vi "CAPTH-Config.vi"(0 "Datafile":path, 5 "Params":T1={"Stimulus"={"EAR"=enum."RIGHT", "HI FREQ"=18.0, "LO FREQ"=5.0, "FREQ STEP"=8, "Rep Rate (/s)"=20.0, "Alternate Polarity"=TRUE, "# CYCLES"=1, "Duration (ms)"=0.0, "Ramp (ms)"=0.0}, "Response"={"Averages (3dB steps)"=12, "Time Window (ms)"=8.5, "dt (us)"=10.0, "Grass gain"=1000.0, "CRITERION (mV)"=60.0, "CEILING (dB atten)"=6.0, "Use previous"=FALSE, "Save avgs"=FALSE, "Save raw"=FALSE, "Save history"=FALSE, "CEILING (dB SPL)"=6.0}} {"Response"."CRITERION (mV)" format="%.2f"; "Response"."Time Window (ms)" format="%.2f"}, 11 "error in (no error)":errorcluster) -> (3 "IO channels":cluster{"Output":u16, "Input":u16}[](array[cluster]), 4 "Freqs":dbl[](array[numeric]), 6 "runtime":T5, 12 "data":T4(array[cluster]), 13 "active ears":i32[](array[numeric]), 14 "start atten":dbl[](array[numeric]), 15 "error out":errorcluster)   [LabVIEW 2020]
uses:
  Typedefs/CAPTH-Runtime.ctl
  Typedefs/CAPTH-Parameters.ctl
  Typedefs/CAPTH-Stimulus.ctl
  Typedefs/CAPTH-Response.ctl
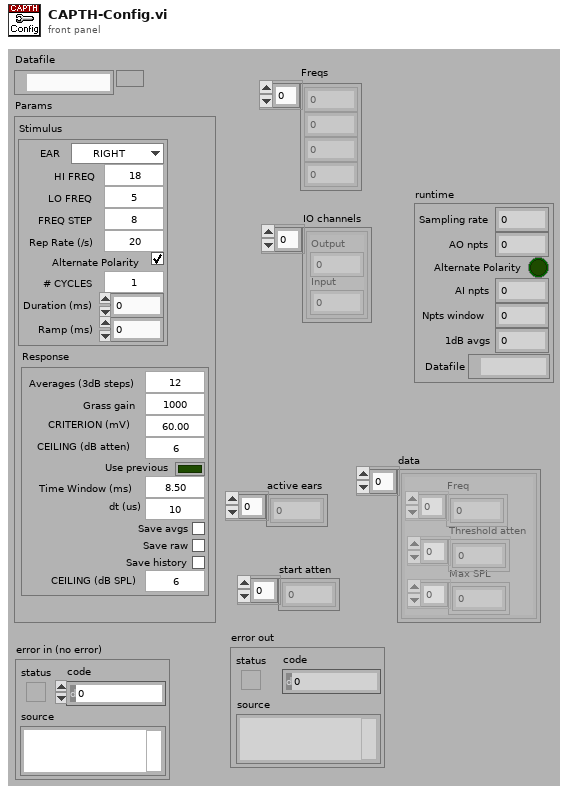
[diagram p1: front panel]
types:
  T1 = typedef "CAPTH-Parameters.ctl" = cluster{"Stimulus":T2, "Response":T3}
  T2 = typedef "CAPTH-Stimulus.ctl" = cluster{"EAR":enum16{"RIGHT", "LEFT\n", "ALTERNATE"}, "HI FREQ":dbl, "LO FREQ":dbl, "FREQ STEP":u8, "Rep Rate (/s)":dbl, "Alternate Polarity":bool, "# CYCLES":u8, "Duration (ms)":dbl, "Ramp (ms)":dbl}
  T3 = typedef "CAPTH-Response.ctl" = cluster{"Averages (3dB steps)":i32, "Time Window (ms)":dbl, "dt (us)":dbl, "Grass gain":dbl, "CRITERION (mV)":dbl, "CEILING (dB atten)":dbl, "Use previous":bool, "Save avgs":bool, "Save raw":bool, "Save history":bool, "CEILING (dB SPL)":dbl}
  T4 = cluster{"Freq":dbl[], "Threshold atten":dbl[], "Max SPL":dbl[]}[]
  T5 = typedef "CAPTH-Runtime.ctl" = cluster{"Sampling rate":dbl, "AO npts":i32, "Alternate Polarity":bool, "AI npts":i32, "Npts window":i32, "1dB avgs":i32, "Datafile":path}
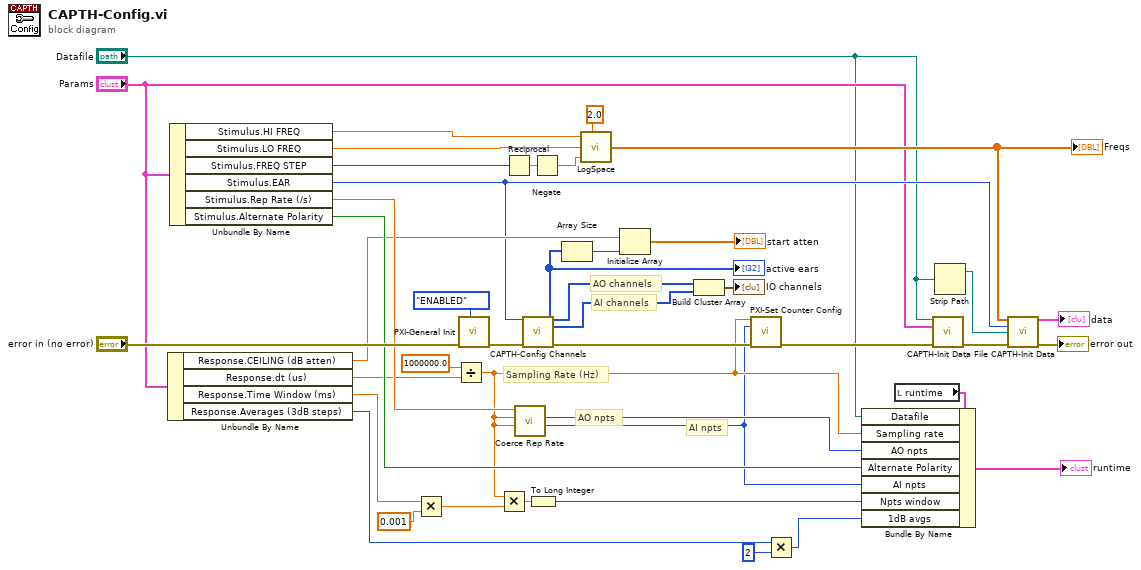
[diagram p0: block diagram]
diagram:
  # "AO channels"
  # "AI channels"
  # "Sampling Rate (Hz)"
  # "AO npts"
  # "AI npts"
  n1 = Unbundle By Name("Params") -> ("Response.CEILING (dB atten)"=w19:dbl, "Response.dt (us)"=w22:dbl, "Response.Time Window (ms)"=w26:dbl, "Response.Averages (3dB steps)"=w27:i32)
  n2 = Unbundle By Name("Params") -> ("Stimulus.HI FREQ"=w34:dbl, "Stimulus.LO FREQ"=w33:dbl, "Stimulus.FREQ STEP"=w32:u8, "Stimulus.EAR"=w15:enum16{"RIGHT", "LEFT\n", "ALTERNATE"}, "Stimulus.Rep Rate (/s)"=w31:dbl, "Stimulus.Alternate Polarity"=w30:bool)
  n3 = Multiply(x=w26, y=0.001) -> (x*y=w24:dbl)
  n4 = Divide(x=1000000.0, y=w22) -> (x/y=w10:dbl)
  n5 = call "PXI-General Init.vi"("Double Buffer Mode"=enum32{"OFF", "ENABLED", "FORCED"}."ENABLED", "error in (no error)"="error in (no error)") -> ("error out"=w38:errorcluster)  [unwired: 9 in]
  n6 = Multiply(x=w10, y=w24) -> (x*y=w23:dbl)
  n7 = Reciprocal(x=w32) -> (1/x=w41:dbl)
  n8 = call "Coerce Rep Rate.vi"("AI sampling rate (Hz)"=w10, "AO sampling rate (Hz)"=w10, "Rep rate (Hz)"=w31) -> ("AI npts"=w4:i32, "AO npts"=w29:i32)  [unwired: 5 in, 2 out]
  n9 = call "CAPTH-Config Channels.vi"("EAR"=w15, "error in (no error)"=w38) -> ("active ears"=w21:i32[], "AO channels"=w37:u16[], "AI channels"=w36:u16[], "error out"=w12:errorcluster)  [unwired: 10 in]
  "active ears" <- w21
  n10 = To Long Integer(number=w23) -> (32bit integer=w5:i32)
  n11 = Negate(x=w41) -> (-x=w39:dbl)
  n12 = Array Size(array=w21) -> (size(s)=w20:i32)
  n13 = call "LogSpace.vi"("Start"=w34, "Base"=2.0, "Stop"=w33, "Step"=w39) -> ("Array"=w16:dbl[])  [unwired: 2 in, 1 out]
  "Freqs" <- w16
  n14 = Initialize Array(w19, w20) -> (→"start atten":dbl[])
  n15 = Build Cluster Array(w37, w36) -> (→"IO channels":cluster{"Left primary":u16, "Right CAP":u16}[])
  n16 = call "PXI-Set Counter Config.vi"("AI Sampling Rate (Hz)"=w10, "Num AI Pts"=w4, "error in (no error)"=w12) -> ("error out"=w11:errorcluster)  [unwired: 12 in]
  n17 = Multiply(x=w27, y=2) -> (x*y=w3:i32)
  n18 = local read "runtime"() -> (w7:T5)
  n19 = Bundle By Name(cluster=w7, "Datafile"="Datafile", "Sampling rate"=w10, "AO npts"=w29, "Alternate Polarity"=w30, "AI npts"=w4, "Npts window"=w5, "1dB avgs"=w3) -> (→"runtime":T5)
  n20 = call "CAPTH-Init Data File.vi"("Datafile path"="Datafile", "Params"="Params", "error in (no error)"=w11) -> ("error out"=w13:errorcluster)  [unwired: 12 in]
  n21 = Strip Path(path="Datafile") -> (stripped path=w8:path)  [unwired: 1 out]
  n22 = call "CAPTH-Init Data.vi"("Freqs"=w16, "EAR"=w15, "Folder"=w8, "error in (no error)"=w13) -> ("data array"=→"data":cluster{"Freqs":dbl[], dbl[], "Max SPL":dbl[]}[], "error out"=→"error out":errorcluster)  [unwired: 10 in]
